vi "testTranformation.vi"() -> ()   [LabVIEW 2009]
uses:
  Hal/Channels/Camera/Camera/Camera.lvclass
  Tools/Filing/FileSystem/FileSystem.lvclass
  Tools/CameraSettings/CamaraSettings.lvclass
  Tools/Filing/FileNeologist/FileNeologist.lvclass
panel:
  in  "saveImages?":bool=TRUE
  in  "number":i32=1
  out "temperature":dbl
  in  "stop":bool
  out "imageSaved":bool
  out "stopped":bool
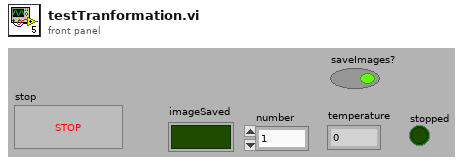
[diagram p1: front panel]
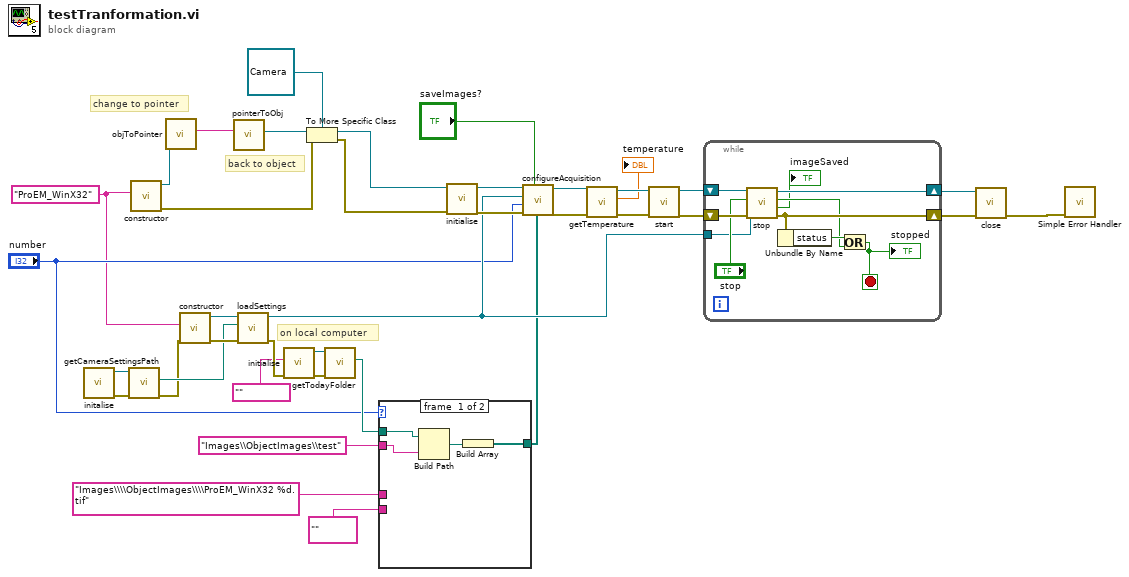
[diagram p0: block diagram]
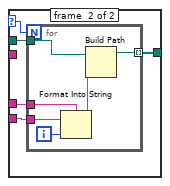
[diagram p2: hidden frame]
diagram:
  w5 = "ProEM_WinX32" ("Camera")
  # "back to object"
  # "change to pointer"
  # "on local computer"
  n1 = call "initalise.vi"() -> ("error out"=w24:errorcluster, "FileSystem out"=w25:refnum<class "FileSystem.lvclass">)  [unwired: 10 in]
  n2 = call-dynamic "getCameraSettingsPath.vi"("error in (no error)"=w24, "FileSystem.lvclass in"=w25) -> ("error out"=w22:errorcluster, "CameraSettingsPath"=w23:path)  [unwired: 7 in, 1 out]
  n3 = call "constructor.vi"("Camera"=w5) -> ("error out"=w2:errorcluster, "Camera out"=w38:refnum<class "Camera.lvclass">)  [unwired: 9 in]
  n4 = call "objToPointer.vi"("objIn"=w38) -> ("stringOut"=w37:string)  [unwired: 10 in]
  n5 = call "constructor.vi"("error in (no error)"=w22, "camera settings"=w5) -> ("error out"=w26:errorcluster, "CamaraSettings out"=w27:refnum<class "CamaraSettings.lvclass">)  [unwired: 8 in]
  n6 = call "pointerToObj.vi"("stringIn"=w37) -> ("objOut"=w36:refnum<class>)  [unwired: 10 in]
  n7 = call-dynamic "loadSettings.vi"("error in (no error)"=w26, "Path"=w23, "CamaraSettings in"=w27) -> ("error out"=w20:errorcluster, "CamaraSettings out"=w21:refnum<class "CamaraSettings.lvclass">)  [unwired: 7 in]
  n8 = call "initialise.vi"("error in (no error)"=w20, "computer name"="") -> ("error out"=w18:errorcluster, "FileNeologist out"=w19:refnum<class "FileNeologist.lvclass">)  [unwired: 8 in]
  n9 = To More Specific Class(target class=refnum<class "Camera.lvclass"> refnum ("Camera out"), reference=w36, error in=w2) -> (specific class reference=w4:refnum<class "Camera.lvclass">, error out=w3:errorcluster)
  n10 = call "getTodayFolder.vi"("error in (no error)"=w18, "FileNeologist in"=w19) -> ("todayFolder"=w11:path)  [unwired: 7 in, 2 out]
  n11 = case shown="-1" "number" {
    selector: "number" -> [_ w44]
    tunnel: w11 -> [w41 w47]
    tunnel: [w42 w46] -> w6
    tunnel: "Images\\\\ObjectImages\\\\ProEM_WinX32 %d.tif" -> [_ w45]
    tunnel: "" -> [_ w43]
    tunnel: "Images\\ObjectImages\\test" -> [w40 _]
    frame #0 {
      n12 = Build Path(base path=w41, name or relative path=w40) -> (appended path=w39:path)
      n13 = Build Array(w39) -> (w42:path[])
    }
    frame #1 {
      n14 = for {
        N: w44 -> [_]
        tunnel: w47 -> [w53]
        tunnel: [w52] -> w46 mode=indexing
        tunnel: w45 -> [w50]
        tunnel: w43 -> [w48]
        i -> [w51]
        n15 = Format Into String(format string=w50, initial string=w48, w51) -> (resulting string=w49:string)  [unwired: 1 in, 1 out]
        n16 = Build Path(base path=w53, name or relative path=w49) -> (appended path=w52:path)
      }
    }
  }
  n17 = call-dynamic "initialise.vi"("error in (no error)"=w3, "Camera in"=w4) -> ("error out"=w28:errorcluster, "Camera out"=w34:refnum<class "Camera.lvclass">)  [unwired: 8 in]
  n18 = call-dynamic "configureAcquisition.vi"("imagePaths"=w6, "saveImages?"="saveImages?", "error in (no error)"=w28, "number of Images"="number", "CameraSettings"=w21, "Camera in"=w34) -> ("error out"=w29:errorcluster, "Camera out"=w33:refnum<class "Camera.lvclass">)  [unwired: 4 in]
  n19 = call-dynamic "getTemperature.vi"("error in (no error)"=w29, "Camera in"=w33) -> ("error out"=w14:errorcluster, "temperature"=→"temperature":dbl, "Camera out"=w32:refnum<class "Camera.lvclass">)  [unwired: 7 in]
  n20 = call-dynamic "start.vi"("error in (no error)"=w14, "Camera in"=w32) -> ("error out"=w30:errorcluster, "Camera out"=w31:refnum<class "Camera.lvclass">)  [unwired: 8 in]
  n21 = while {
    tunnel: w21 -> [w59]
    shift-right: [w62] -> w15
    shift-left: w31 -> [w63]
    shift-right: [w58] -> w16
    shift-left: w30 -> [w61]
    stop <- w55 stop-if-true
    n22 = call-dynamic "stop.vi"("error in (no error)"=w61, "CameraSettings"=w59, "stop"="stop", "Camera in"=w63) -> ("error out"=w58:errorcluster, "imageSaved"=→"imageSaved":bool, "stopped?"=w56:bool, "Camera out"=w62:refnum<class "Camera.lvclass">)  [unwired: 4 in]
    n23 = Unbundle By Name(w58) -> ("status"=w57:bool)
    n24 = Or(x=w57, y=w56) -> (x .or. y?=w55:bool)
    "stopped" <- w55
  }
  n25 = call-dynamic "close.vi"("error in (no error)"=w16, "Camera in"=w15) -> ("error out"=w13:errorcluster)  [unwired: 9 in]
  n26 = call <vilib>:"Simple Error Handler.vi"("error in (no error)"=w13) -> ()  [unwired: 4 in, 5 out]
